vi "Equivalent Circuits Parameters.vi"(8 "error in (no error)":errorcluster, 11 "VISA resource name":refnum<visa-resource-name>) -> (0 "error out":errorcluster, 1 "Ca [F]":dbl format="%^.3e", 2 "L [H]":dbl format="%^.3e", 3 "VISA resource name out":refnum<visa-resource-name>, 4 "Cb [F]":dbl format="%^.3e", 5 "R [ohm]":dbl format="%^.3e")   [LabVIEW 2017, in "Agilent 4194.lvlib"]
doc: "This function outputs the equivalent circuits R, L, Ca, Cb parameters data."
uses:
  Agilent 4194.lvlib
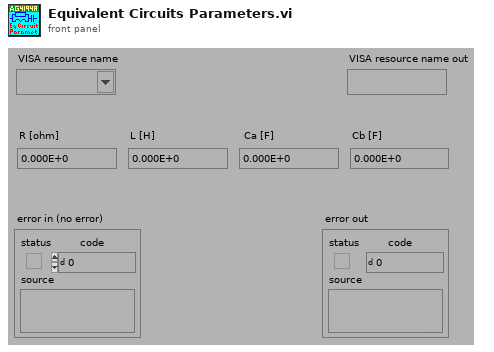
[diagram p1: front panel]
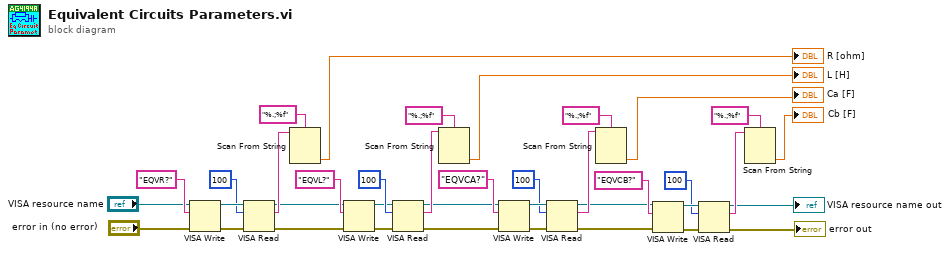
[diagram p0: block diagram]
diagram:
  n1 = VISA Write(VISA resource name="VISA resource name", write buffer="EQVR?" ("write buffer (\"\")"), error in (no error)="error in (no error)") -> (VISA resource name out=w32:refnum<visa-resource-name>, error out=w33:errorcluster)  [unwired: 1 out]
  n2 = VISA Read(VISA resource name=w32, byte count=u32 100 ("byte count (0)"), error in (no error)=w33) -> (VISA resource name out=w17:refnum<visa-resource-name>, read buffer=w29:string, error out=w16:errorcluster)  [unwired: 1 out]
  n3 = Scan From String(format string="%.;%f", input string=w29) -> (output 1=→"R [ohm]":dbl)  [unwired: 3 in, 3 out]
  n4 = VISA Write(VISA resource name=w17, write buffer="EQVL?" ("write buffer (\"\")"), error in (no error)=w16) -> (VISA resource name out=w25:refnum<visa-resource-name>, error out=w24:errorcluster)  [unwired: 1 out]
  n5 = VISA Read(VISA resource name=w25, byte count=u32 100 ("byte count (0)"), error in (no error)=w24) -> (VISA resource name out=w15:refnum<visa-resource-name>, read buffer=w27:string, error out=w14:errorcluster)  [unwired: 1 out]
  n6 = Scan From String(format string="%.;%f", input string=w27) -> (output 1=→"L [H]":dbl)  [unwired: 3 in, 3 out]
  n7 = VISA Write(VISA resource name=w15, write buffer="EQVCA?" ("write buffer (\"\")"), error in (no error)=w14) -> (VISA resource name out=w22:refnum<visa-resource-name>, error out=w23:errorcluster)  [unwired: 1 out]
  n8 = VISA Read(VISA resource name=w22, byte count=u32 100 ("byte count (0)"), error in (no error)=w23) -> (VISA resource name out=w11:refnum<visa-resource-name>, read buffer=w20:string, error out=w10:errorcluster)  [unwired: 1 out]
  n9 = Scan From String(format string="%.;%f", input string=w20) -> (output 1=→"Ca [F]":dbl)  [unwired: 3 in, 3 out]
  n10 = VISA Write(VISA resource name=w11, write buffer="EQVCB?" ("write buffer (\"\")"), error in (no error)=w10) -> (VISA resource name out=w37:refnum<visa-resource-name>, error out=w38:errorcluster)  [unwired: 1 out]
  n11 = VISA Read(VISA resource name=w37, byte count=u32 100 ("byte count (0)"), error in (no error)=w38) -> (VISA resource name out=→"VISA resource name out":refnum<visa-resource-name>, read buffer=w34:string, error out=→"error out":errorcluster)  [unwired: 1 out]
  n12 = Scan From String(format string="%.;%f", input string=w34) -> (output 1=→"Cb [F]":dbl)  [unwired: 3 in, 3 out]
